vi "connectPubDataPublish.vi"(8 "error in (no error)":errorcluster, 11 "MiddlewareSVThisComponent in":refnum<class "MiddlewareSVThisComponent.lvclass">) -> (0 "error out":errorcluster, 3 "MiddlewareSVThisComponent out":refnum<class "MiddlewareSVThisComponent.lvclass">)   [LabVIEW 2016, in "MiddlewareSVThisComponent.lvclass"]
uses:
  MiddlewareSVThisComponent.lvclass
  ConfigurationTC/ConfigurationTypedefs/Base/CommunicationConfig.ctl
  ConfigurationTC/ConfigurationTypedefs/ConfigurationTypedefs.lvlib
  ConfigurationTC/ConfigurationTypedefs/Base/SVProcessConfig.ctl
  Typedefs/PubDataSV.ctl
  Typedefs/EXATypedefs.lvlib
  <vilib>/Utility/Data Type/NI_Data Type.lvlib
  ComponentTemplateCore/ComponentModel/ComponentModel/ConfigurationFileReader/ConfigurationFileReader.lvclass
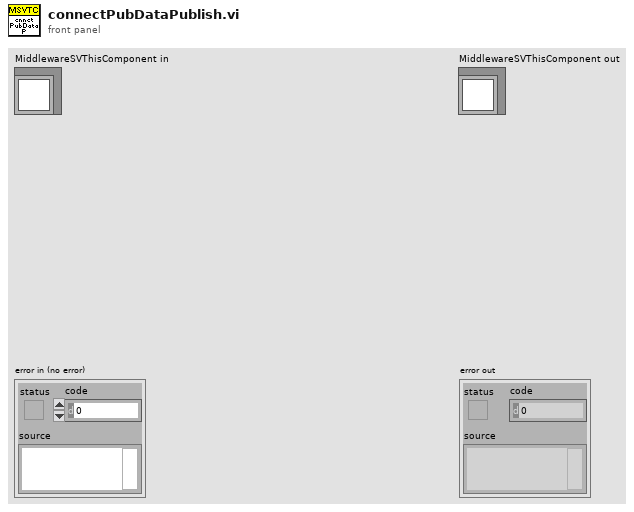
[diagram p1: front panel]
types:
  T1 = typedef "ConfigurationTypedefs.lvlib/SVProcessConfig.ctl" = cluster{"subDataProcessPrototype":string, "pubDataProcessPrototype":string, "commandProcessPrototype":string, "commandSVName":string}
  T2 = typedef "EXATypedefs.lvlib/PubDataSV.ctl" = enum16{"DetailedState", "ErrorCode", "Heartbeat", "LoopTime_ms", "LoopTimeOutOfRange", "RejectedCommand", "SummaryState", "Timestamp", "SettingVersions", "SettingsApplied", "AppliedSettingsMatchStart"}
  T3 = typedef "ConfigurationTypedefs.lvlib/CommunicationConfig.ctl" = cluster{"hostComputerAddress":string, "ComponentAcronym":string, "InstanceIdentifier":i32}
  T4 = cluster{"Read Access":enum8{"Allowed", "Required", "None"}, "Write Access":enum8{"Allowed", "Required", "None"}}
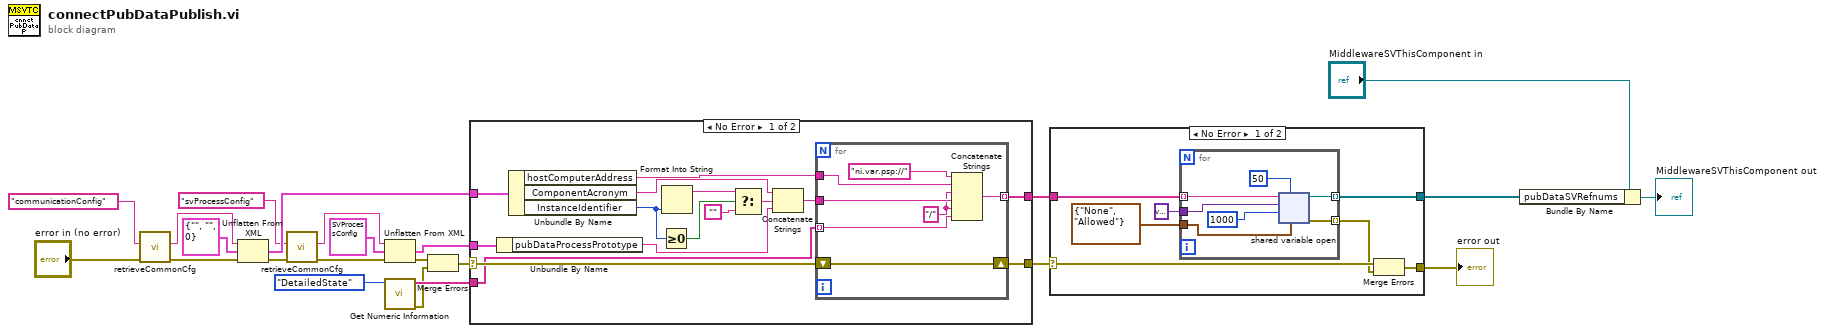
[diagram p0: block diagram]
diagram:
  n1 = call "retrieveCommonCfg.vi"("error in (no error)"="error in (no error)", "dataName"="communicationConfig") -> ("error out"=w5:errorcluster, "dataValueFromFile"=w6:string)  [unwired: 7 in, 1 out]
  n2 = Unflatten From XML(xml string=w6, type=T3 {"hostComputerAddress"="", "ComponentAcronym"="", "InstanceIdentifier"=0} ("sharedVariableLibrariesConfig"), error in (no error)=w5) -> (value=w17:T3, error out=w4:errorcluster)
  n3 = call "retrieveCommonCfg.vi"("error in (no error)"=w4, "dataName"="svProcessConfig") -> ("error out"=w3:errorcluster, "dataValueFromFile"=w2:string)  [unwired: 7 in, 1 out]
  n4 = Unflatten From XML(xml string=w2, type=T1 {"subDataProcessPrototype"="SubDataSV", "pubDataProcessPrototype"="PubDataSV", "commandProcessPrototype"="CommandSV", "commandSVName"="Command"} ("svProcessConfig"), error in (no error)=w3) -> (value=w15:T1, error out=w16:errorcluster)
  n5 = call <vilib>:"Get Numeric Information.vi"("Variant"=PubDataSV."DetailedState" ("PubDataSV")) -> ("error out"=w12:errorcluster, "Enum Names"=w13:string[])  [unwired: 7 in, 2 out]
  n6 = Merge Errors(w16, w12) -> (w19:errorcluster)
  n7 = case shown="No Error" w19 {
    selector: w19 -> [w33 w46]
    tunnel: [w38 _] -> w21
    tunnel: w17 -> [w36 _]
    tunnel: [w32 w46] -> w22
    tunnel: w13 -> [w26 _]
    tunnel: w15 -> [w25 _]
    frame No Error {
      n8 = Unbundle By Name(w25) -> ("pubDataProcessPrototype"=w24:string)
      n9 = Unbundle By Name(w36) -> ("hostComputerAddress"=w35:string, "ComponentAcronym"=w37:string, "InstanceIdentifier"=w31:i32)
      n10 = Greater Or Equal To 0?(x=w31) -> (x >= 0?=w30:bool)
      n11 = Format Into String(w31) -> (resulting string=w29:string)  [unwired: 3 in, 1 out]
      n12 = Select(t=w29, s=w30, f="") -> (s? t:f=w27:string)
      n13 = Concatenate Strings(w37, w27, w24) -> (w34:string)
      n14 = for {
        tunnel: w35 -> [w44]
        tunnel: w34 -> [w43]
        tunnel: [w41] -> w38 mode=indexing
        shift-right: [w39] -> w32
        shift-left: w33 -> [w39]
        tunnel: w26 -> [w40] mode=indexing
        w42 = "/" ("string")
        n15 = Concatenate Strings("ni.var.psp://" ("string"), w44, w42, w43, w42, w40) -> (w41:string)
      }
    }
    frame Error {
    }
  }
  n16 = case shown="No Error" w22 {
    selector: w22 -> [w51 w61]
    tunnel: w21 -> [w52 _]
    tunnel: [w48 w61] -> w10
    tunnel: [w47 _] -> w20
    frame No Error {
      n17 = for {
        tunnel: T4 {"Read Access"=enum."None", "Write Access"=enum."Allowed"} ("access") -> [w60]
        tunnel: w52 -> [w59] mode=indexing
        tunnel: [w57] -> w47 mode=indexing
        tunnel: variant ("variant") -> [w56]
        tunnel: [w58] -> w50 mode=indexing
        n18 = shared-variable-open(w59, w56, w60, 1000 ("timeout ms"), u32 50 ("buffer size in elements")) -> (w57:refnum<k21>, w58:errorcluster)  [unwired: 1 in]
      }
      n19 = Merge Errors(w51, w50) -> (w48:errorcluster)
    }
    frame Error {
    }
  }
  "error out" <- w10
  n20 = Bundle By Name(cluster="MiddlewareSVThisComponent in", "pubDataSVRefnums"=w20) -> (→"MiddlewareSVThisComponent out":refnum<class "MiddlewareSVThisComponent.lvclass">)
